vi "GetLimsTestStep.vi"(8 "error in (no error)":errorcluster, 10 "Step-id":i32, 11 "ByteGSAPIBase in":refnum<class "ByteGSAPIBase.lvclass">) -> (0 "error out":errorcluster, 2 "StepList":T1, 3 "ByteGSAPIBase out":refnum<class "ByteGSAPIBase.lvclass">)   [LabVIEW 2019, in "ByteGSWebAPI.lvlib" / "ByteGSAPIBase.lvclass"]
doc: "Get a single Step based on Step-Id"
uses:
  ByteGSAPIBase.lvclass
  TypeDef/Step.ctl
  TypeDef/Asset.ctl
  ByteGSAPIBase.lvclass/ByteGSAPIBase.ctl
  <vilib>/Bytelabs/ByteREST/ByteRESTClass/ByteRESTBase/RESTBase.lvclass
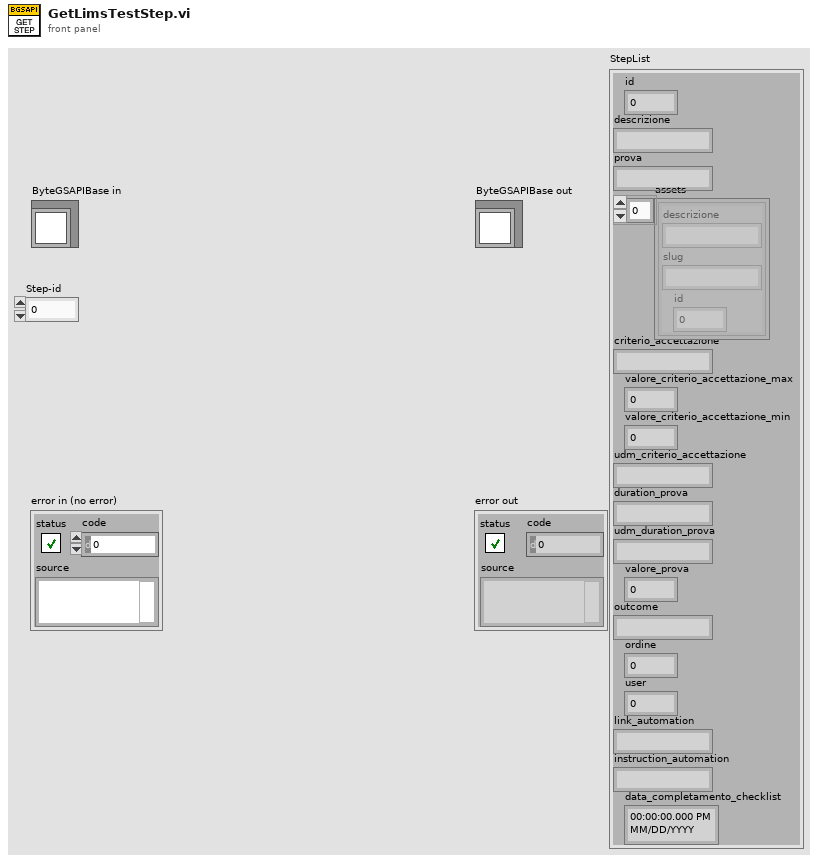
[diagram p1: front panel]
types:
  T1 = typedef "ByteGSWebAPI.lvlib/ByteGSAPIBase.lvclass/Step.ctl" = cluster{"id":i32, "descrizione":string, "prova":string, "assets":T2[], "criterio_accettazione":string, "valore_criterio_accettazione_max":dbl, "valore_criterio_accettazione_min":dbl, "udm_criterio_accettazione":string, "duration_prova":string, "udm_duration_prova":string, "valore_prova":dbl, "outcome":string, "ordine":i32, "user":i32, "link_automation":string, "instruction_automation":string, "data_completamento_checklist":timestamp}
  T2 = typedef "ByteGSWebAPI.lvlib/ByteGSAPIBase.lvclass/Asset.ctl" = cluster{"descrizione":string, "slug":string, "id":i32}
  T3 = cluster{"id":i32, "descrizione":string, "prova":string, "assets":T2[], "criterio_accettazione":string, "valore_criterio_accettazione_max":dbl, "valore_criterio_accettazione_min":dbl, "udm_criterio_accettazione":string, "duration_prova":string, "udm_duration_prova":string, "data_completamento_checklist":string, "valore_prova":dbl, "outcome":string, "ordine":i32, "user":i32, "link_automation":string, "instruction_automation":string}[]
  T4 = cluster{"id":i32, "descrizione":string, "prova":string, "assets":T2[], "criterio_accettazione":string, "valore_criterio_accettazione_max":dbl, "valore_criterio_accettazione_min":dbl, "udm_criterio_accettazione":string, "duration_prova":string, "udm_duration_prova":string, "data_completamento_checklist":string, "valore_prova":dbl, "outcome":string, "ordine":i32, "user":i32, "link_automation":string, "instruction_automation":string}
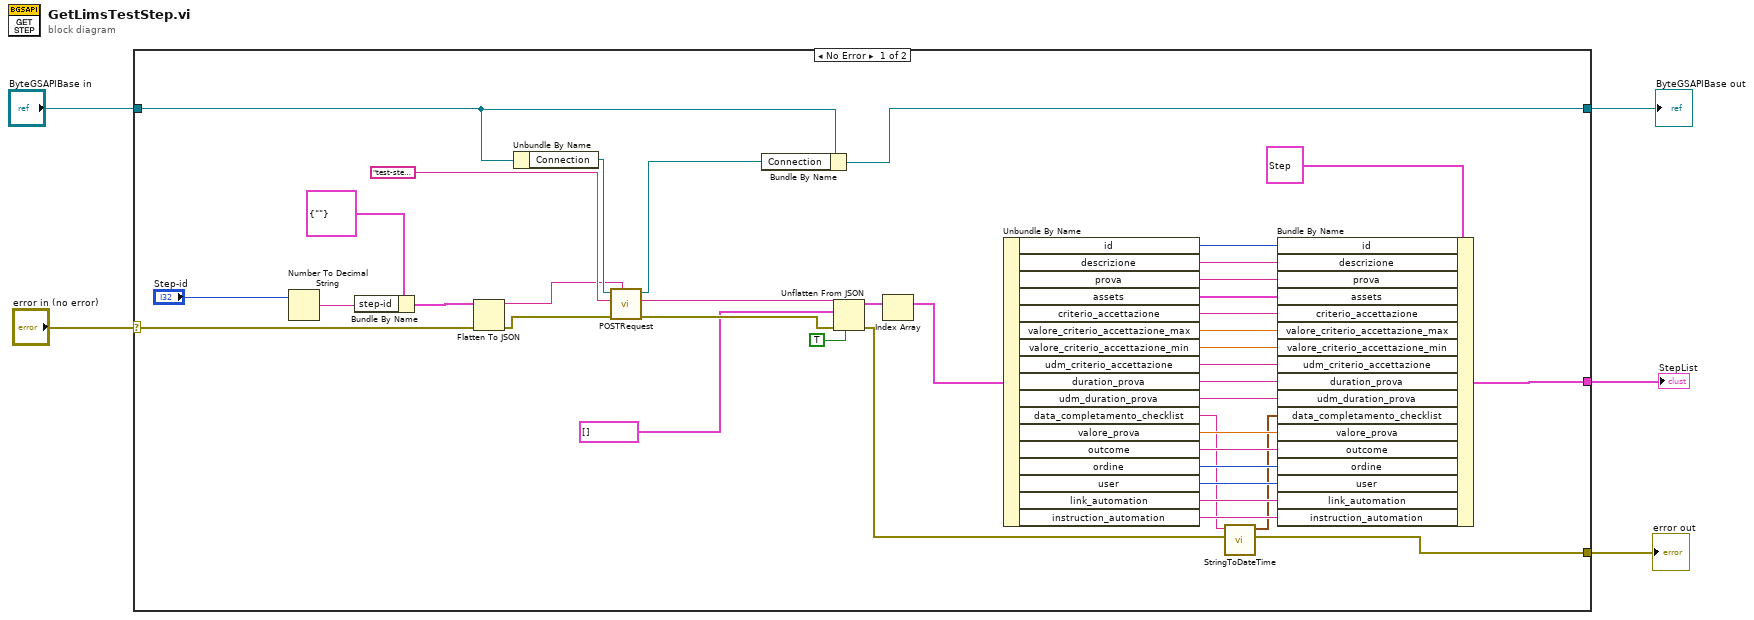
[diagram p0: block diagram]
diagram:
  n1 = case shown="No Error" "error in (no error)" {
    selector: "error in (no error)" -> [w35 w47]
    tunnel: [w13 w47] -> w4
    tunnel: [w42 w46] -> w2
    tunnel: "ByteGSAPIBase in" -> [w43 w46]
    tunnel: [w10 _] -> w1
    frame No Error {
      n2 = Number To Decimal String(number="Step-id") -> (decimal integer string=w39:string)  [unwired: 1 in]
      n3 = Bundle By Name(cluster=cluster{"step-id":string} {"step-id"=""} ("Request"), "step-id"=w39) -> (w37:cluster{"step-id":string})
      n4 = Flatten To JSON(anything=w37, error in (no error)=w35) -> (JSON string=w36:string, 11:w34:errorcluster)  [unwired: 1 in]
      n5 = Unbundle By Name(w43) -> ("Connection"=w45:refnum<class "RESTBase.lvclass">)
      n6 = call-dynamic "POSTRequest.vi"("Body in"=w36, "error in (no error)"=w34, "Request"="test-step-list", "ByteRESTBase in"=w45) -> ("error out"=w32:errorcluster, "Body"=w33:string, "ByteRESTBase out"=w44:refnum<class "RESTBase.lvclass">)  [unwired: 4 in, 1 out]
      n7 = Bundle By Name(cluster=w43, "Connection"=w44) -> (w42:refnum<class "ByteGSAPIBase.lvclass">)
      n8 = Unflatten From JSON(JSON string=w33, type and defaults=T3 [], default null elements? (F)=TRUE, error in (no error)=w32) -> (value=w7:T3, error out=w12:errorcluster)  [unwired: 3 in]
      n9 = Index Array(array=w7) -> (element=w8:T4)  [unwired: 1 in]
      n10 = Unbundle By Name(w8) -> ("id"=w14:i32, "descrizione"=w15:string, "prova"=w16:string, "assets"=w17:T2[], "criterio_accettazione"=w18:string, "valore_criterio_accettazione_max"=w19:dbl, "valore_criterio_accettazione_min"=w20:dbl, "udm_criterio_accettazione"=w21:string, "duration_prova"=w22:string, "udm_duration_prova"=w23:string, "data_completamento_checklist"=w24:string, "valore_prova"=w26:dbl, "outcome"=w27:string, "ordine"=w28:i32, "user"=w29:i32, "link_automation"=w30:string, "instruction_automation"=w31:string)
      n11 = call "StringToDateTime.vi"("error in (no error)"=w12, "datetime string"=w24) -> ("error out"=w13:errorcluster, "timestamp"=w25:timestamp)  [unwired: 8 in]
      n12 = Bundle By Name(cluster=T1 {"id"=0, "descrizione"="", "prova"="", "assets"=[], "criterio_accettazione"="", "valore_criterio_accettazione_max"=0.0, "valore_criterio_accettazione_min"=0.0, "udm_criterio_accettazione"="", "duration_prova"="", "udm_duration_prova"="", "valore_prova"=0.0, "outcome"="", "ordine"=0, "user"=0, "link_automation"="", "instruction_automation"="", "data_completamento_checklist"=timestamp(0 s since 1904-01-01)} ("StepList"), "id"=w14, "descrizione"=w15, "prova"=w16, "assets"=w17, "criterio_accettazione"=w18, "valore_criterio_accettazione_max"=w19, "valore_criterio_accettazione_min"=w20, "udm_criterio_accettazione"=w21, "duration_prova"=w22, "udm_duration_prova"=w23, "data_completamento_checklist"=w25, "valore_prova"=w26, "outcome"=w27, "ordine"=w28, "user"=w29, "link_automation"=w30, "instruction_automation"=w31) -> (w10:T1)
    }
    frame Error {
    }
  }
  "error out" <- w4
  "ByteGSAPIBase out" <- w2
  "StepList" <- w1
